vi "电缸控制 - 副本.vi"() -> ()   [LabVIEW 2014]
uses:
  <vilib>/Utility/error.llb/DialogType.ctl
  <vilib>/DAQmx/create/channels.llb/DAQmx Create Channel (DI-Digital Input).vi
  <vilib>/DAQmx/read.llb/DAQmx Read (Digital 1D Bool 1Chan 1Samp).vi
  <vilib>/DAQmx/create/channels.llb/DAQmx Create Channel (DO-Digital Output).vi
  <vilib>/DAQmx/write.llb/DAQmx Write (Digital 1D Bool 1Chan 1Samp).vi
panel:
  in  "输出设备":tag
  in  "输入设备":tag
  in  "初始化":bool
  in  "停止":bool
  in  "复位":bool
  in  "步序号":u32
  in  "定位运转":bool
  in  "步信息":T1
  in  "返回原点":bool
  out "控制器输入":T2
  in  "人工输出":T3
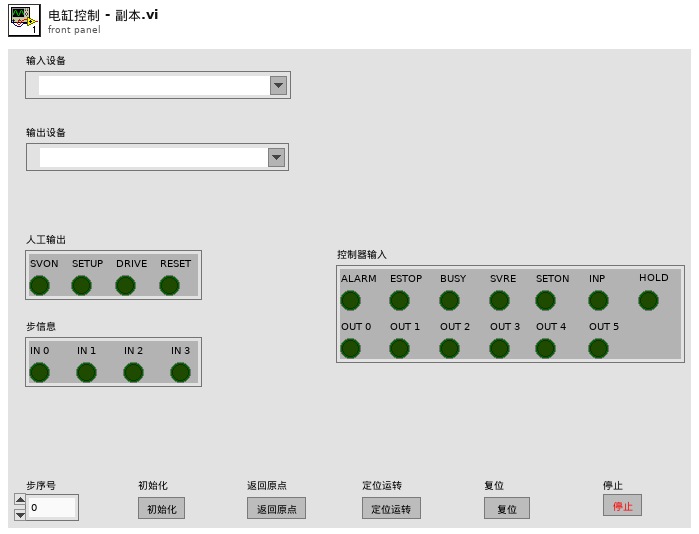
[diagram p1: front panel]
types:
  T1 = cluster{"IN 0":bool, "IN 1":bool, "IN 2":bool, "IN 3":bool}
  T2 = cluster{"ALARM":bool, "ESTOP":bool, "BUSY":bool, "SVRE":bool, "SETON":bool, "INP":bool, "HOLD":bool, "OUT 0":bool, "OUT 1":bool, "OUT 2":bool, "OUT 3":bool, "OUT 4":bool, "OUT 5":bool}
  T3 = cluster{"SVON":bool, "SETUP":bool, "DRIVE":bool, "RESET":bool}
  T4 = typedef "DialogType.ctl" = u16
  T5 = cluster{"data[0]":bool, "data[1]":bool, "data[2]":bool, "data[3]":bool, "data[4]":bool, "data[5]":bool, "data[6]":bool, "data[7]":bool, "data[8]":bool, "data[9]":bool, "data[10]":bool, "data[11]":bool, "data[12]":bool}
  T6 = cluster{"Boolean array[0]":bool, "Boolean array[1]":bool, "Boolean array[2]":bool, "Boolean array[3]":bool}
  T7 = cluster{"Boolean array[0]":bool, "Boolean array[1]":bool, "Boolean array[2]":bool, "Boolean array[3]":bool, "Boolean array[4]":bool, "Boolean array[5]":bool, "Boolean array[6]":bool, "Boolean array[7]":bool, "Boolean array[8]":bool, "Boolean array[9]":bool, "Boolean array[10]":bool, "Boolean array[11]":bool, "Boolean array[12]":bool}
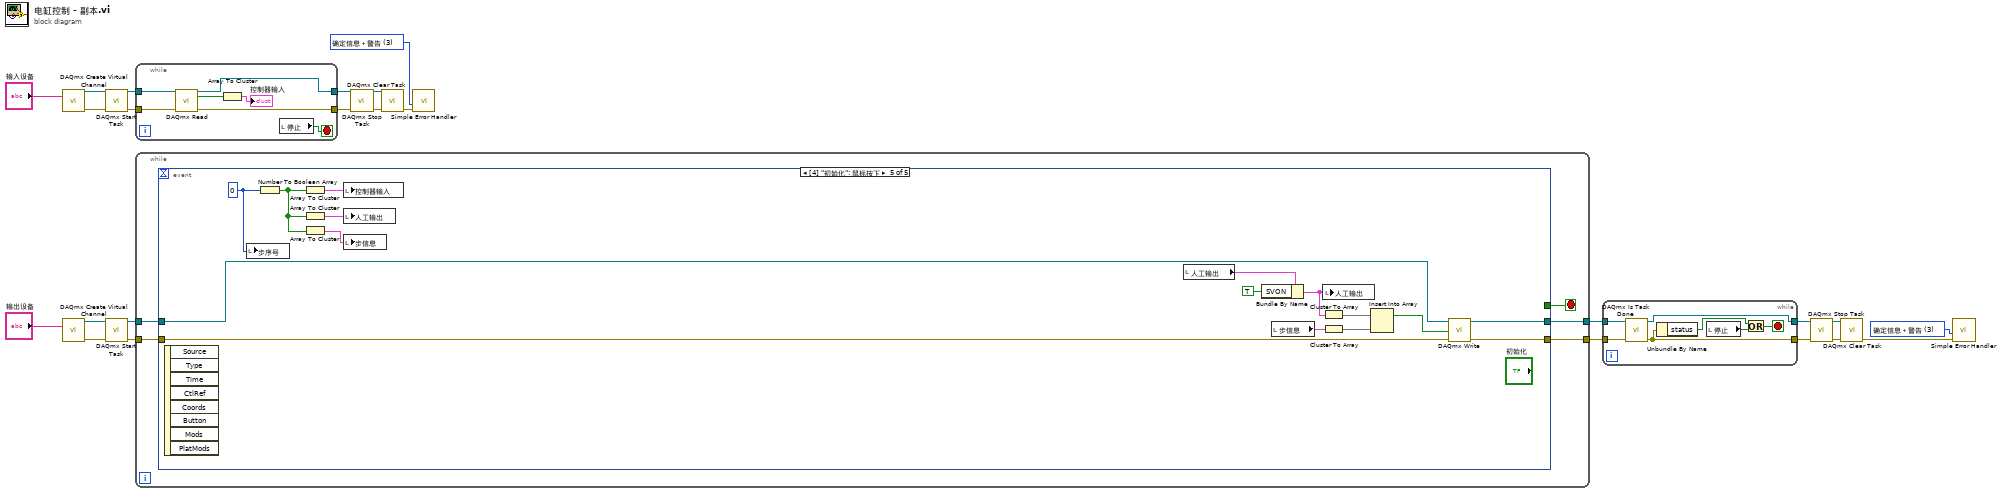
[diagram p0: block diagram]
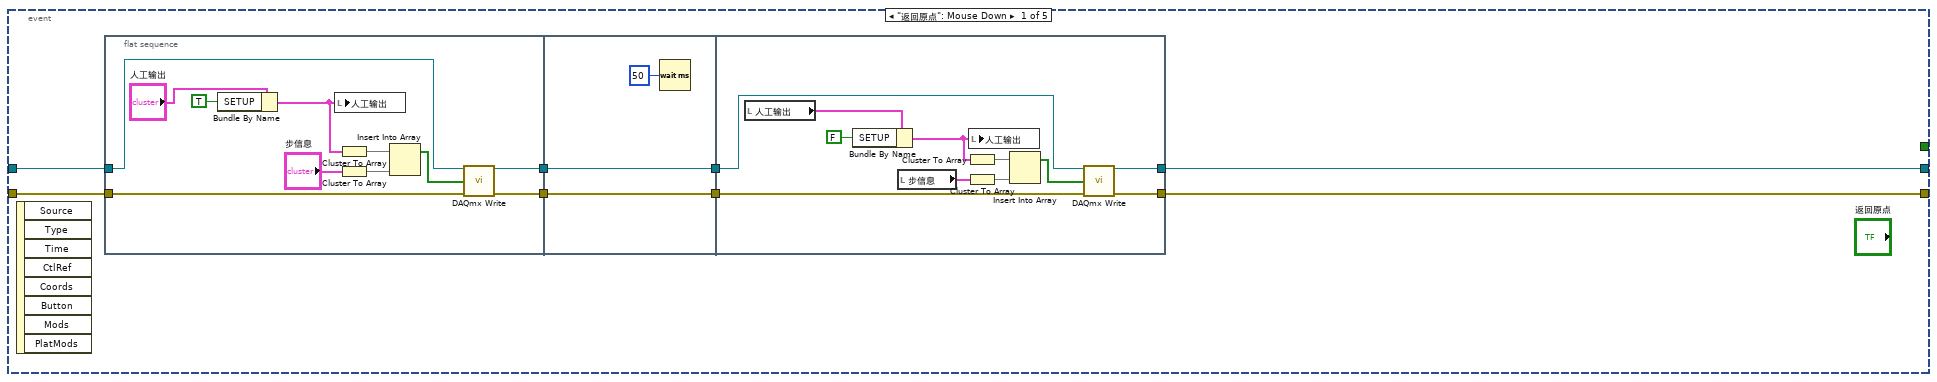
[diagram p2: hidden frame]
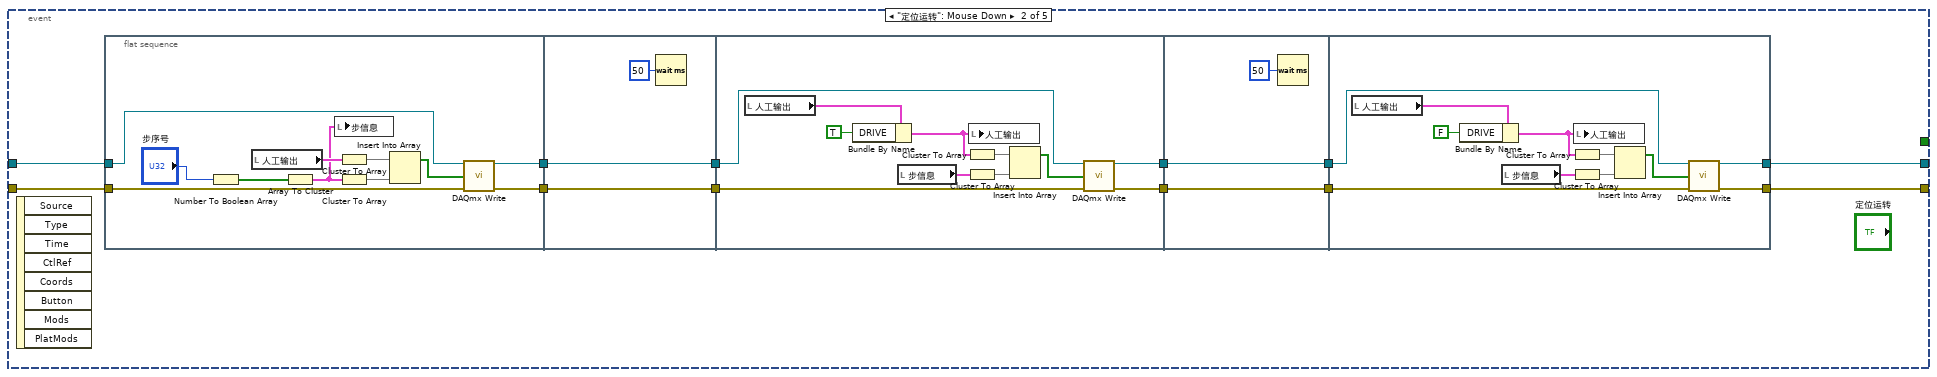
[diagram p3: hidden frame]
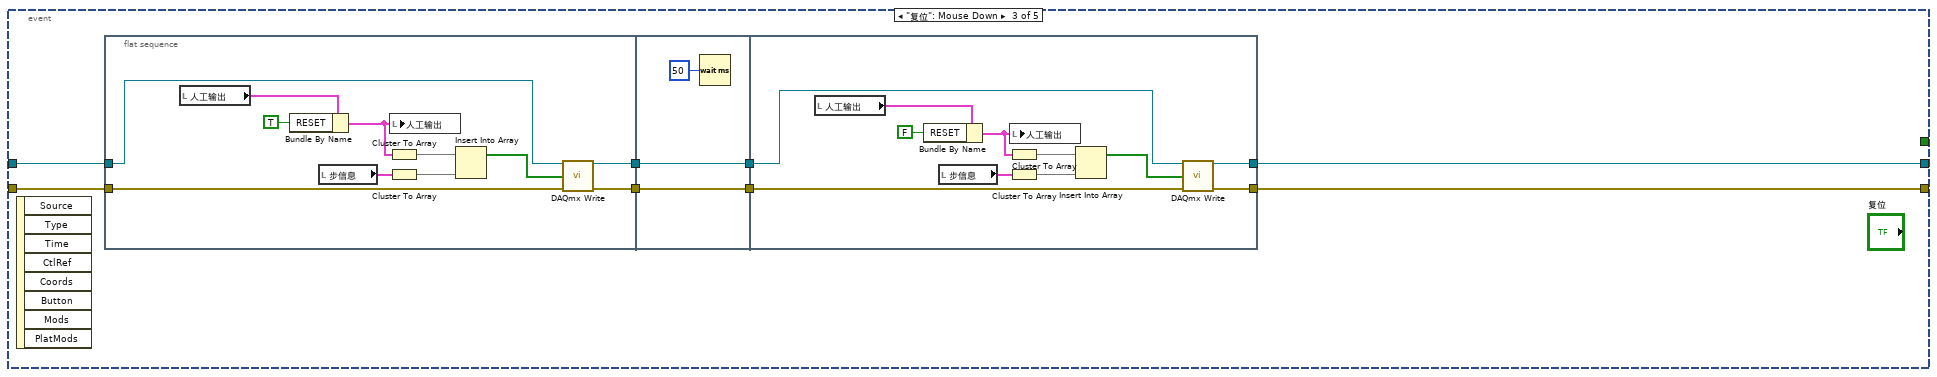
[diagram p4: hidden frame]
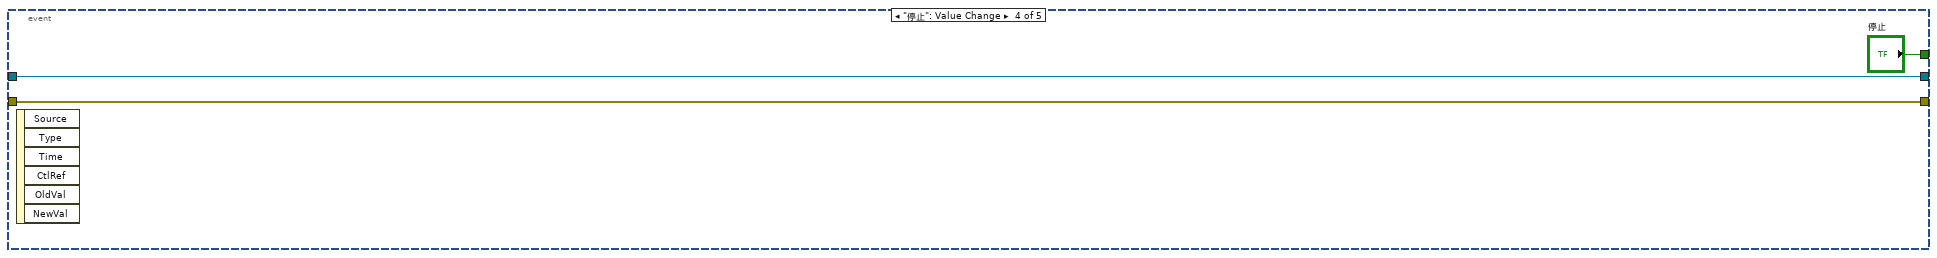
[diagram p5: hidden frame]
diagram:
  w1 = T4 3 items=["无对话框", "确定信息", "继续或停止信息", "确定信息＋警告", "继续/停止+警告"] ("type of dialog (OK msg:1)")
  w16 = T4 3 items=["无对话框", "确定信息", "继续或停止信息", "确定信息＋警告", "继续/停止+警告"] ("type of dialog (OK msg:1)")
  n1 = call-poly <vilib>:"DAQmx Create Virtual Channel.vi"("lines"="输入设备") -> ("task out"=w15:refnum<k21>, "error out"=w14:errorcluster)  [unwired: 13 in]
  n2 = call-poly <vilib>:"DAQmx Create Virtual Channel.vi"("lines"="输出设备") -> ("task out"=w12:refnum<k21>, "error out"=w13:errorcluster)  [unwired: 13 in]
  n3 = call <vilib>:"DAQmx Start Task.vi"("task/channels in"=w15, "error in"=w14) -> ("task out"=w23:refnum<k21>, "error out"=w22:errorcluster)  [unwired: 12 in]
  n4 = call <vilib>:"DAQmx Start Task.vi"("task/channels in"=w12, "error in"=w13) -> ("task out"=w10:refnum<k21>, "error out"=w9:errorcluster)  [unwired: 12 in]
  n5 = while {
    tunnel: w23 -> [w30]
    tunnel: w22 -> [w29]
    tunnel: [w28] -> w21
    tunnel: [w27] -> w20
    stop <- w31 stop-if-true
    n6 = call-poly <vilib>:"DAQmx Read.vi"("task/channels in"=w30, "error in"=w29) -> ("task out"=w28:refnum<k21>, "data"=w26:bool[], "error out"=w27:errorcluster)  [unwired: 11 in]
    n7 = Array To Cluster(array=w26) -> (cluster=→"控制器输入":T5)
    n8 = local read "停止"() -> (w31:bool)
  }
  n9 = while {
    tunnel: w10 -> [w35]
    tunnel: w9 -> [w34]
    tunnel: [w33] -> w8
    tunnel: [w32] -> w7
    stop <- w36 stop-if-true
    n10 = event shown="[4] \"初始化\": 鼠标按下" {
      selector: _ -> [_ _ _ _ _]
      dyn-events: _ -> [_ _ _ _ _]
      timeout: _ -> [_ _ _ _ _]
      tunnel: [_ _ _ "停止" _] -> w36
      tunnel: w35 -> [w38 w81 w124 w155 w162]
      tunnel: w34 -> [w37 w80 w123 w154 w161]
      tunnel: [w40 w71 w122 w155 w160] -> w33
      tunnel: [w39 w70 w121 w154 w159] -> w32
      event "返回原点": Mouse Down {
        n11 = event-data() -> ()  [unwired: 1 in, 8 out]
        n12 = flat-sequence {
          tunnel: [w50] -> w44
          tunnel: [w49] -> w41
          tunnel: w38 -> [w48]
          tunnel: w37 -> [w47]
          tunnel: w44 -> [w58]
          tunnel: [w58] -> w43
          tunnel: [w57] -> w42
          tunnel: w41 -> [w57]
          tunnel: w43 -> [w62]
          tunnel: w42 -> [w61]
          tunnel: [w60] -> w40
          tunnel: [w59] -> w39
          frame #0 {
            n13 = Bundle By Name(cluster="人工输出", "SETUP"=TRUE) -> (w54:T3)
            n14 = local write "人工输出"(w54) -> ()
            n15 = Cluster To Array(cluster=w54) -> (array=w53:bool[])
            n16 = Cluster To Array(cluster="步信息") -> (array=w52:bool[])
            n17 = Insert Into Array(array=w53, new element=w52) -> (w51:bool[])  [unwired: 1 in]
            n18 = call-poly <vilib>:"DAQmx Write.vi"("task/channels in"=w48, "data"=w51, "error in"=w47) -> ("task out"=w50:refnum<k21>, "error out"=w49:errorcluster)  [unwired: 10 in, 1 out]
          }
          frame #1 {
            n19 = Wait (ms)(milliseconds to wait=u32 50 ("等待时间（毫秒）")) -> ()  [unwired: 1 out]
          }
          frame #2 {
            n20 = local read "人工输出"() -> (w69:T3)
            n21 = Bundle By Name(cluster=w69, "SETUP"=FALSE) -> (w67:T3)
            n22 = local read "步信息"() -> (w66:T1)
            n23 = Cluster To Array(cluster=w67) -> (array=w65:bool[])
            n24 = Cluster To Array(cluster=w66) -> (array=w64:bool[])
            n25 = local write "人工输出"(w67) -> ()
            n26 = Insert Into Array(array=w65, new element=w64) -> (w63:bool[])  [unwired: 1 in]
            n27 = call-poly <vilib>:"DAQmx Write.vi"("task/channels in"=w62, "data"=w63, "error in"=w61) -> ("task out"=w60:refnum<k21>, "error out"=w59:errorcluster)  [unwired: 10 in, 1 out]
          }
        }
      }
      event "定位运转": Mouse Down {
        n28 = event-data() -> ()  [unwired: 1 in, 8 out]
        n29 = flat-sequence {
          tunnel: w81 -> [w88]
          tunnel: w80 -> [w87]
          tunnel: [w85] -> w79
          tunnel: [w84] -> w76
          tunnel: w79 -> [w95]
          tunnel: [w95] -> w78
          tunnel: [w94] -> w77
          tunnel: w76 -> [w94]
          tunnel: w78 -> [w99]
          tunnel: w77 -> [w98]
          tunnel: [w97] -> w74
          tunnel: [w96] -> w72
          tunnel: [w109] -> w75
          tunnel: w74 -> [w109]
          tunnel: [w108] -> w73
          tunnel: w72 -> [w108]
          tunnel: w75 -> [w118]
          tunnel: w73 -> [w117]
          tunnel: [w111] -> w71
          tunnel: [w110] -> w70
          frame #0 {
            n30 = Number To Boolean Array(number="步序号") -> (Boolean array=w89:bool[])
            n31 = local read "人工输出"() -> (w91:T3)
            n32 = Array To Cluster(array=w89) -> (cluster=w83:T6)
            n33 = local write "步信息"(w83) -> ()
            n34 = Cluster To Array(cluster=w91) -> (array=w90:bool[])
            n35 = Cluster To Array(cluster=w83) -> (array=w82:bool[])
            n36 = Insert Into Array(array=w90, new element=w82) -> (w86:bool[])  [unwired: 1 in]
            n37 = call-poly <vilib>:"DAQmx Write.vi"("task/channels in"=w88, "data"=w86, "error in"=w87) -> ("task out"=w85:refnum<k21>, "error out"=w84:errorcluster)  [unwired: 10 in, 1 out]
          }
          frame #1 {
            n38 = Wait (ms)(milliseconds to wait=u32 50 ("毫秒倍数")) -> ()  [unwired: 1 out]
          }
          frame #2 {
            n39 = local read "人工输出"() -> (w106:T3)
            n40 = Bundle By Name(cluster=w106, "DRIVE"=TRUE) -> (w104:T3)
            n41 = local read "步信息"() -> (w103:T1)
            n42 = Cluster To Array(cluster=w104) -> (array=w102:bool[])
            n43 = Cluster To Array(cluster=w103) -> (array=w101:bool[])
            n44 = local write "人工输出"(w104) -> ()
            n45 = Insert Into Array(array=w102, new element=w101) -> (w100:bool[])  [unwired: 1 in]
            n46 = call-poly <vilib>:"DAQmx Write.vi"("task/channels in"=w99, "data"=w100, "error in"=w98) -> ("task out"=w97:refnum<k21>, "error out"=w96:errorcluster)  [unwired: 10 in, 1 out]
          }
          frame #3 {
            n47 = Wait (ms)(milliseconds to wait=u32 50 ("毫秒倍数")) -> ()  [unwired: 1 out]
          }
          frame #4 {
            n48 = local read "人工输出"() -> (w120:T3)
            n49 = Bundle By Name(cluster=w120, "DRIVE"=FALSE) -> (w116:T3)
            n50 = local read "步信息"() -> (w115:T1)
            n51 = Cluster To Array(cluster=w116) -> (array=w114:bool[])
            n52 = Cluster To Array(cluster=w115) -> (array=w113:bool[])
            n53 = local write "人工输出"(w116) -> ()
            n54 = Insert Into Array(array=w114, new element=w113) -> (w112:bool[])  [unwired: 1 in]
            n55 = call-poly <vilib>:"DAQmx Write.vi"("task/channels in"=w118, "data"=w112, "error in"=w117) -> ("task out"=w111:refnum<k21>, "error out"=w110:errorcluster)  [unwired: 10 in, 1 out]
          }
        }
      }
      event "复位": Mouse Down {
        n56 = event-data() -> ()  [unwired: 1 in, 8 out]
        n57 = flat-sequence {
          tunnel: w124 -> [w133]
          tunnel: w123 -> [w132]
          tunnel: [w130] -> w127
          tunnel: [w129] -> w125
          tunnel: [w142] -> w128
          tunnel: w127 -> [w142]
          tunnel: [w141] -> w126
          tunnel: w125 -> [w141]
          tunnel: w128 -> [w147]
          tunnel: w126 -> [w146]
          tunnel: [w144] -> w122
          tunnel: [w143] -> w121
          frame #0 {
            n58 = local read "人工输出"() -> (w139:T3)
            n59 = Bundle By Name(cluster=w139, "RESET"=TRUE ("HOLD")) -> (w137:T3)
            n60 = local read "步信息"() -> (w136:T1)
            n61 = Cluster To Array(cluster=w137) -> (array=w135:bool[])
            n62 = Cluster To Array(cluster=w136) -> (array=w134:bool[])
            n63 = local write "人工输出"(w137) -> ()
            n64 = Insert Into Array(array=w135, new element=w134) -> (w131:bool[])  [unwired: 1 in]
            n65 = call-poly <vilib>:"DAQmx Write.vi"("task/channels in"=w133, "data"=w131, "error in"=w132) -> ("task out"=w130:refnum<k21>, "error out"=w129:errorcluster)  [unwired: 10 in, 1 out]
          }
          frame #1 {
            n66 = Wait (ms)(milliseconds to wait=u32 50 ("毫秒倍数")) -> ()  [unwired: 1 out]
          }
          frame #2 {
            n67 = local read "人工输出"() -> (w153:T3)
            n68 = Bundle By Name(cluster=w153, "RESET"=FALSE ("HOLD")) -> (w151:T3)
            n69 = local read "步信息"() -> (w150:T1)
            n70 = Cluster To Array(cluster=w151) -> (array=w149:bool[])
            n71 = Cluster To Array(cluster=w150) -> (array=w148:bool[])
            n72 = local write "人工输出"(w151) -> ()
            n73 = Insert Into Array(array=w149, new element=w148) -> (w145:bool[])  [unwired: 1 in]
            n74 = call-poly <vilib>:"DAQmx Write.vi"("task/channels in"=w147, "data"=w145, "error in"=w146) -> ("task out"=w144:refnum<k21>, "error out"=w143:errorcluster)  [unwired: 10 in, 1 out]
          }
        }
      }
      event "停止": Value Change {
        n75 = event-data() -> ()  [unwired: 1 in, 6 out]
      }
      event "初始化": Mouse Down {
        w157 = u32 0 ("数字")
        n76 = event-data() -> ()  [unwired: 1 in, 8 out]
        n77 = local write "步序号"(w157) -> ()
        n78 = Number To Boolean Array(number=w157) -> (Boolean array=w170:bool[])
        n79 = Array To Cluster(array=w170) -> (cluster=w172:T7)
        n80 = Array To Cluster(array=w170) -> (cluster=w171:T6)
        n81 = Array To Cluster(array=w170) -> (cluster=w169:T6)
        n82 = local write "控制器输入"(w172) -> ()
        n83 = local write "人工输出"(w171) -> ()
        n84 = local write "步信息"(w169) -> ()
        n85 = local read "人工输出"() -> (w168:T3)
        n86 = Bundle By Name(cluster=w168, "SVON"=TRUE) -> (w166:T3)
        n87 = local read "步信息"() -> (w165:T1)
        n88 = Cluster To Array(cluster=w166) -> (array=w164:bool[])
        n89 = Cluster To Array(cluster=w165) -> (array=w163:bool[])
        n90 = local write "人工输出"(w166) -> ()
        n91 = Insert Into Array(array=w164, new element=w163) -> (w158:bool[])  [unwired: 1 in]
        n92 = call-poly <vilib>:"DAQmx Write.vi"("task/channels in"=w162, "data"=w158, "error in"=w161) -> ("task out"=w160:refnum<k21>, "error out"=w159:errorcluster)  [unwired: 10 in, 1 out]
      }
    }
  }
  n93 = call <vilib>:"DAQmx Stop Task.vi"("task/channels in"=w21, "error in"=w20) -> ("task out"=w19:refnum<k21>, "error out"=w18:errorcluster)  [unwired: 12 in]
  n94 = call <vilib>:"DAQmx Clear Task.vi"("task in"=w19, "error in"=w18) -> ("error out"=w17:errorcluster)  [unwired: 13 in]
  n95 = call <vilib>:"Simple Error Handler.vi"("type of dialog (OK msg:1)"=w16, "error in (no error)"=w17) -> ()  [unwired: 3 in, 5 out]
  n96 = while {
    tunnel: w8 -> [w179]
    tunnel: w7 -> [w178]
    tunnel: [w177] -> w6
    tunnel: [w176] -> w5
    stop <- w173 stop-if-true
    n97 = call <vilib>:"DAQmx Is Task Done.vi"("task/channels in"=w179, "error in"=w178) -> ("task out"=w177:refnum<k21>, "error out"=w176:errorcluster)  [unwired: 11 in, 1 out]
    n98 = Unbundle By Name(w176) -> ("status"=w175:bool)
    n99 = local read "停止"() -> (w174:bool)
    n100 = Or(x=w175, y=w174) -> (x .or. y?=w173:bool)
  }
  n101 = call <vilib>:"DAQmx Stop Task.vi"("task/channels in"=w6, "error in"=w5) -> ("task out"=w4:refnum<k21>, "error out"=w3:errorcluster)  [unwired: 12 in]
  n102 = call <vilib>:"DAQmx Clear Task.vi"("task in"=w4, "error in"=w3) -> ("error out"=w2:errorcluster)  [unwired: 13 in]
  n103 = call <vilib>:"Simple Error Handler.vi"("type of dialog (OK msg:1)"=w1, "error in (no error)"=w2) -> ()  [unwired: 3 in, 5 out]
